vi "DLTS - run 2 pulse DAQ (SubVI).vi"(0 "ziModHandle":T2 {"ModHandle" format="0x%08x"; "Conn" format="0x%08x"}, 1 "ziHandle":T1 {"Handle" format="0x%08x"; "Conn" format="0x%08x"}, 2 "pulse length 2":dbl[unit], 3 "Vpulse 2":dbl[unit], 4 "Vbias":dbl[unit], 5 "error in (no error)":errorcluster, 6 "pulse length":dbl[unit], 7 "Timeout":dbl, 8 "Vpulse":dbl[unit], 9 "Averaging":u32, 10 "occurrence":refnum<k4>, 12 "Status string":refnum<vi>) -> (14 "ModHandle Out":T2 {"ModHandle" format="0x%08x"; "Conn" format="0x%08x"}, 15 "t":dbl[](array[numeric]), 16 "Capacitance transient":dbl[](array[numeric]), 19 "error out":errorcluster)   [LabVIEW 2019]
uses:
  <instrlib>/Zurich Instruments LabOne/Public/Modules/ziTypeModHandle.ctl
  <instrlib>/Zurich Instruments LabOne/Zurich Instruments LabOne.lvlib
  <instrlib>/Zurich Instruments LabOne/Public/ziTypeHandle.ctl
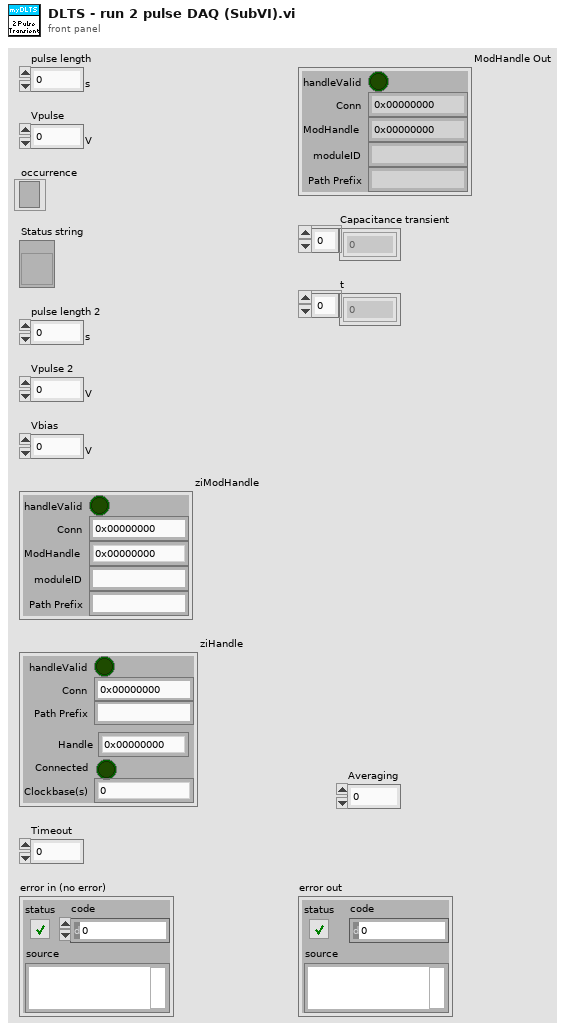
[diagram p1: front panel]
types:
  T1 = typedef "Zurich Instruments LabOne.lvlib/ziTypeHandle.ctl" = cluster{"handleValid":bool, "Conn":u64, "Path Prefix":string, "Handle":u64, "Connected":bool, "Clockbase(s)":dbl}
  T2 = typedef "Zurich Instruments LabOne.lvlib/ziTypeModHandle.ctl" = cluster{"handleValid":bool, "Conn":u64, "ModHandle":u64, "moduleID":string, "Path Prefix":string}
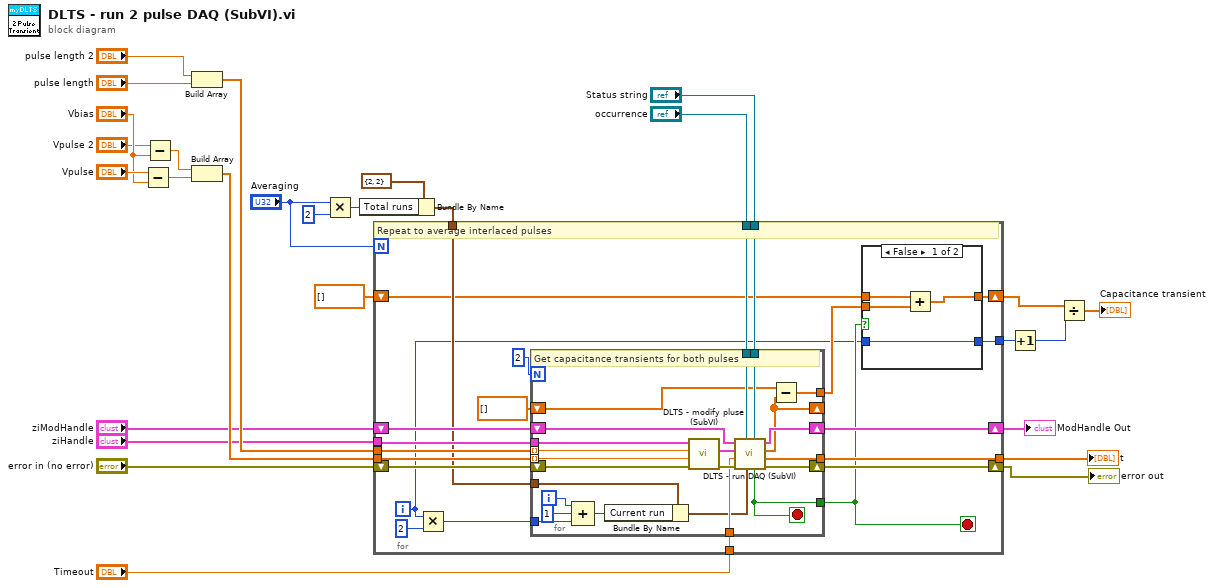
[diagram p0: block diagram]
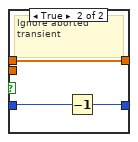
[diagram p2: hidden frame]
diagram:
  n1 = Subtract(x="Vpulse", y="Vbias") -> (x-y=w21:dbl[unit])
  n2 = Subtract(x="Vpulse 2", y="Vbias") -> (x-y=w22:dbl[unit])
  n3 = Build Array("pulse length 2", "pulse length") -> (w23:dbl[unit][])
  n4 = Build Array(w22, w21) -> (w20:dbl[unit][])
  n5 = Multiply(x="Averaging", y=2) -> (x*y=w15:u32)
  n6 = Bundle By Name(cluster=cluster{"Current run":u32, "Total runs":u32} {"Current run"=2, "Total runs"=2} ("Runs"), "Total runs"=w15) -> (w14:cluster{"Current run":u32, "Total runs":u32})
  n7 = for {
    N: "Averaging" -> [_]
    tunnel: w23 -> [w50]
    tunnel: w20 -> [w48]
    tunnel: "Timeout" -> [w47]
    shift-right: [w44] -> w12
    shift-left: "error in (no error)" -> [w45]
    shift-right: [w43] -> w13
    shift-left: "ziModHandle" -> [w42]
    tunnel: "ziHandle" -> [w41]
    tunnel: "occurrence" -> [w40]
    tunnel: "Status string" -> [w39]
    tunnel: w14 -> [w37]
    tunnel: [w36] -> w11
    shift-right: [w33] -> w4
    shift-left: dbl[] [] -> [w32]
    tunnel: [w29] -> w3
    i -> [w30]
    stop <- w31 stop-if-true
    # "Repeat to average interlaced pulses"
    n8 = Multiply(x=w30, y=2) -> (x*y=w38:i32)
    n9 = for {
      N: 2 -> [_]
      tunnel: w41 -> [w78]
      shift-right: [w76] -> w43
      shift-left: w42 -> [w77]
      shift-right: [w74] -> w44
      shift-left: w45 -> [w75]
      tunnel: [w73] -> w36
      tunnel: w39 -> [w72]
      tunnel: w40 -> [w71]
      tunnel: [w70] -> w31
      tunnel: w50 -> [w69] mode=indexing
      tunnel: w48 -> [w68] mode=indexing
      tunnel: w47 -> [w67]
      tunnel: w38 -> [w65]
      tunnel: w37 -> [w61]
      shift-right: [w59] -> _
      shift-left: dbl[] [] ("Samples") -> [w60]
      tunnel: [w58] -> w34
      i -> [w66]
      stop <- w70 stop-if-true
      # "Get capacitance transients for both pulses"
      n10 = Compound Arithmetic op=ADD(w66, 1 ("value"), w65) -> (w63:i32)
      n11 = Bundle By Name(cluster=w61, "Current run"=w63) -> (w62:cluster{"Current run":u32, "Total runs":u32})
      n12 = call "DLTS - modify pluse (SubVI).vi"("error in (no error)"=w75, "AUX scale"=w68, "TUpulse on time"=w69, "Handle Out in"=w78) -> ("error out"=w79:errorcluster, "Handle Out out"=w80:T1)  [unwired: 6 in]
      n13 = call "DLTS - run DAQ (SubVI).vi"("Status String Reference"=w72, "Runs"=w62, "Abort Occurrence"=w71, "error in (no error)"=w79, "Timeout 5000ms"=w67, "Handle in"=w80, "ModHandle in"=w77) -> ("error out"=w74:errorcluster, "t"=w73:dbl[], "Samples"=w59:dbl[], "ModHandle Out  out"=w76:T2, "Aborted"=w70:bool)
      n14 = Subtract(x=w60, y=w59) -> (x-y=w58:dbl[])
    }
    n15 = case shown="False" w31 {
      tunnel: w34 -> [w54 _]
      tunnel: [w53 w57] -> w33
      tunnel: w32 -> [w52 w57]
      tunnel: w30 -> [w51 w56]
      tunnel: [w51 w55] -> w29
      frame False {
        n16 = Add(x=w52, y=w54) -> (x+y=w53:dbl[])
      }
      frame True {
        # "Ignore aborted transient"
        n17 = Decrement(x=w56) -> (x-1=w55:i32)
      }
    }
  }
  "ModHandle Out" <- w13
  "t" <- w11
  "error out" <- w12
  n18 = Increment(x=w3) -> (x+1=w1:i32)
  n19 = Divide(x=w4, y=w1) -> (x/y=→"Capacitance transient":dbl[])
